vi "Get DAQ Scan Timestamp.vi"(7 "Daq Thread":T1, 8 "error in (no error)":errorcluster, 11 "DaqData dCVT":T2) -> (0 "error out":errorcluster, 1 "Time Stamp":timestamp, 2 "Timestamp (DBL)":dbl, 3 "DaqData dCVT out":T2)   [LabVIEW 2017, in "DAQ.lvclass"]
doc: "Developed by Kevin Thompson\nkevin@thompsonengineering.net\n\nCopyright 2018-2020\nThompson Engineering, LLC\nAI scan timestamp is stored with IOName \"%sScanTS\" in DAQ Data Dict\n(%s = ['AI' | 'DI'])"
uses:
  DAQ.lvclass
  <vilib>/TELLC/Dynamic CVT API/TD Dynamic CVT DVR--ref.ctl
  TD DaqThread--enum.ctl
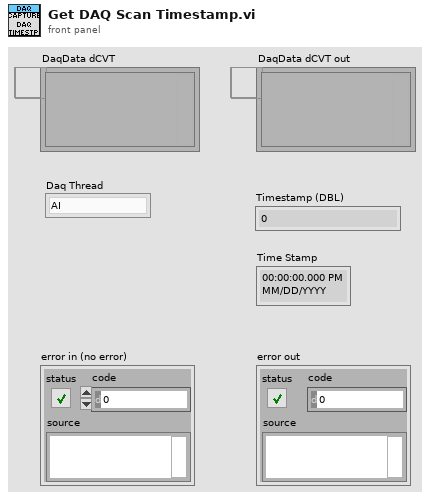
[diagram p1: front panel]
types:
  T1 = typedef "DAQ.lvclass/TD DaqThread--enum.ctl" = enum16{"AI", "DI"}
  T2 = typedef "TD Dynamic CVT DVR--ref.ctl" = refnum<data-value>
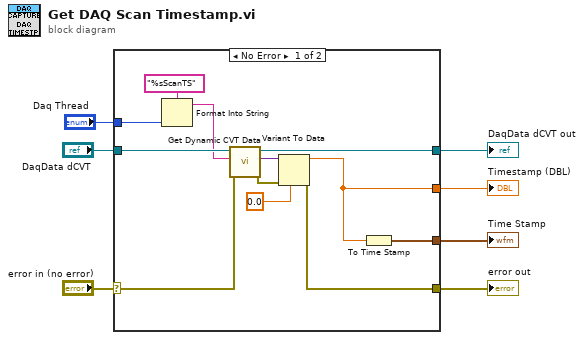
[diagram p0: block diagram]
diagram:
  n1 = case shown="No Error" "error in (no error)" {
    selector: "error in (no error)" -> [w17 w20]
    tunnel: [w11 w20] -> w7
    tunnel: [w19 w21] -> w6
    tunnel: "DaqData dCVT" -> [w18 w21]
    tunnel: [w9 _] -> w3
    tunnel: "Daq Thread" -> [w16 _]
    tunnel: [w8 _] -> w1
    frame No Error {
      n2 = Format Into String(format string="%sScanTS" ("initial string"), w16) -> (resulting string=w14:string)  [unwired: 2 in, 1 out]
      n3 = call <vilib>:"Get Dynamic CVT Data.vi"("error in (no error)"=w17, "DataName"=w14, "dCVT DVR"=w18) -> ("error out"=w12:errorcluster, "value"=w13:variant, "dCVT DVR out"=w19:T2)  [unwired: 5 in, 1 out]
      n4 = Variant To Data(error in=w12, type=0.0, Variant=w13) -> (data=w9:dbl, error out=w11:errorcluster)
      n5 = To Time Stamp(1:w9) -> (0:w8:timestamp)
    }
    frame Error {
    }
  }
  "error out" <- w7
  "DaqData dCVT out" <- w6
  "Timestamp (DBL)" <- w3
  "Time Stamp" <- w1
